vi "tutorial 4.vi"() -> ()   [LabVIEW 2022 SP3]
panel:
  out "Read Meassage":string
  in  "function name":string
  in  "Python version":string
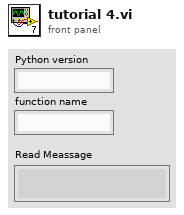
[diagram p1: front panel]
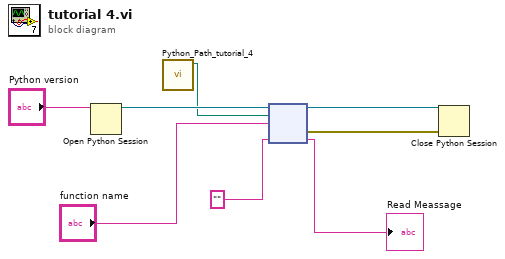
[diagram p0: block diagram]
diagram:
  n1 = Open Python Session(python version="Python version") -> (session out=w7:refnum<k35>)  [unwired: 2 in, 1 out]
  n2 = call "Python_Path_tutorial_4.vi"() -> ("appended path"=w4:path)  [unwired: 11 in]
  n3 = node(w7, w4, "function name", "") -> (w6:refnum<k35>, w5:errorcluster, →"Read Meassage":string)  [unwired: 1 in, 2 out]
  n4 = Close Python Session(session in=w6, error in=w5) -> ()  [unwired: 1 out]
